vi "Unsupported Function Warning.vi"(8 "error in":errorcluster, 10 "Unsupported Function":string, 11 "Acopian in":refnum<class "Acopian.lvclass">) -> (0 "error out":errorcluster, 3 "Acopian out":refnum<class "Acopian.lvclass">)   [LabVIEW 2019, in "Acopian.lvlib" / "Acopian.lvclass"]
uses:
  Library/Acopian.lvclass
  C:/Users/Public/Documents/Development/builds/Instruments/Instruments.lvlibp/Library/Instruments.lvclass
  builds/Instruments/Instruments.lvlibp/Accessors/Generate Warning.vi
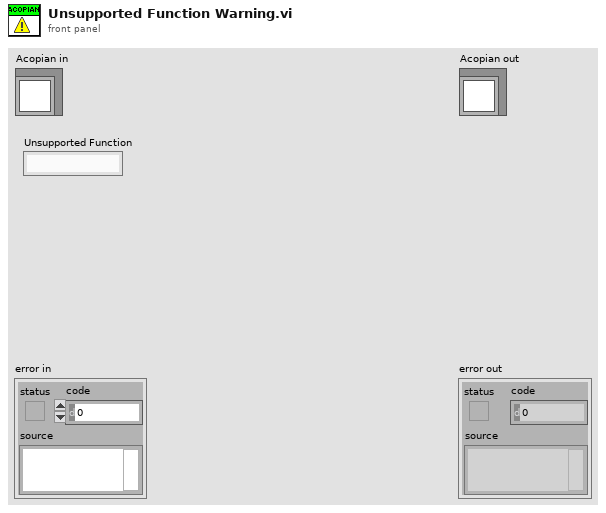
[diagram p1: front panel]
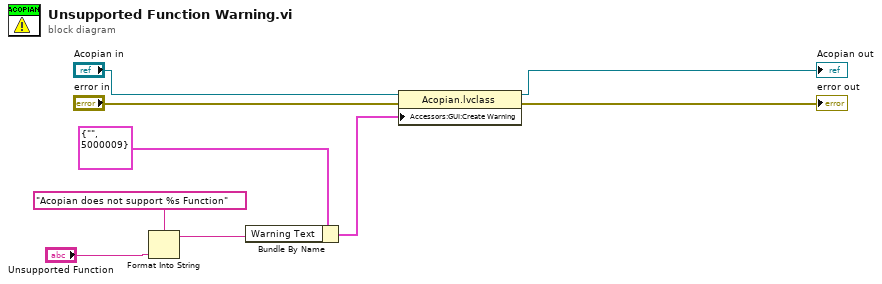
[diagram p0: block diagram]
diagram:
  n1 = Format Into String(format string="Acopian does not support %s Function", "Unsupported Function") -> (resulting string=w2:string)  [unwired: 2 in, 1 out]
  n2 = Bundle By Name(cluster=cluster{"Warning Text":string, "code":i32} {"Warning Text"="", "code"=5000009} ("Instrument:GUI:Create Warning"), "Warning Text"=w2) -> (w3:cluster{"Warning Text":string, "code":i32})
  n3 = property class="Acopian.lvclass"(reference="Acopian in", error in="error in", "Accessors:GUI:Create Warning"=w3) -> (reference out=→"Acopian out":refnum<class "Acopian.lvclass">, error out=→"error out":errorcluster)
